vi "DB - [CMS].[Config].[WindowView].vi"(0 "connection reference":T3, 1 "DB Connection":T4={"Open"=TRUE, "Close"=TRUE}, 2 "DB - CMS Config View":T2, 3 "<Values>":string[](array[string])=["Seq 1/2: +150°C/hr to 80°C"], 5 "DB.Schema.Table\nCMS.Config.View":string="CMS.Config.View", 9 "[PlantId],[StationId]":T1, 11 "error in (no error)":errorcluster) -> (4 "connection reference":T3, 6 "data":string[][](array[string]), 15 "SUMMARY":errorcluster)   [LabVIEW 2013]
uses:
  <vilib>/addons/database/Connection.llb/Conn ObjectReference.ctl
  Controls/DB - OpenClose.ctl
  Controls/DB - CMS Config WindowView.ctl
  Controls/Global SRTRS.vi
  Controls/Global CMS.vi
  <vilib>/addons/database/Connection.llb/DB Tools Open Connec (String).vi
  <vilib>/addons/database/Connection.llb/Conn Execute.vi
  <vilib>/addons/database/Recordset.llb/Rec Fetch Recordset Data (R).vi
  <vilib>/addons/database/Recordset.llb/Rec Destroy - Connection.vi
  <vilib>/addons/database/NI_Database_API.lvlib
panel:
  in  "DB.Schema.Table\nCMS.Config.Station":string="CMS.Config.Station"
  out "Close":errorcluster
  out "SQL Statement":string
  in  "DB.Schema.Table \nCMS.Config.WindowView":string="CMS.Config.WindowView"
  out "CMS Connection Information":T5={"Connection "="SQL Server 32bit HPEnvy", "Username"="admin", "Password"="admin123"}
  # "2014-10-21 15:01\n[TabId],                         w.[No],        v.[ToggleTabInterval],w.[ToggleWinInterval], v.[ToggleTab],        v.[DisplayPlant],       w.[Window01],            w.[Window02]"
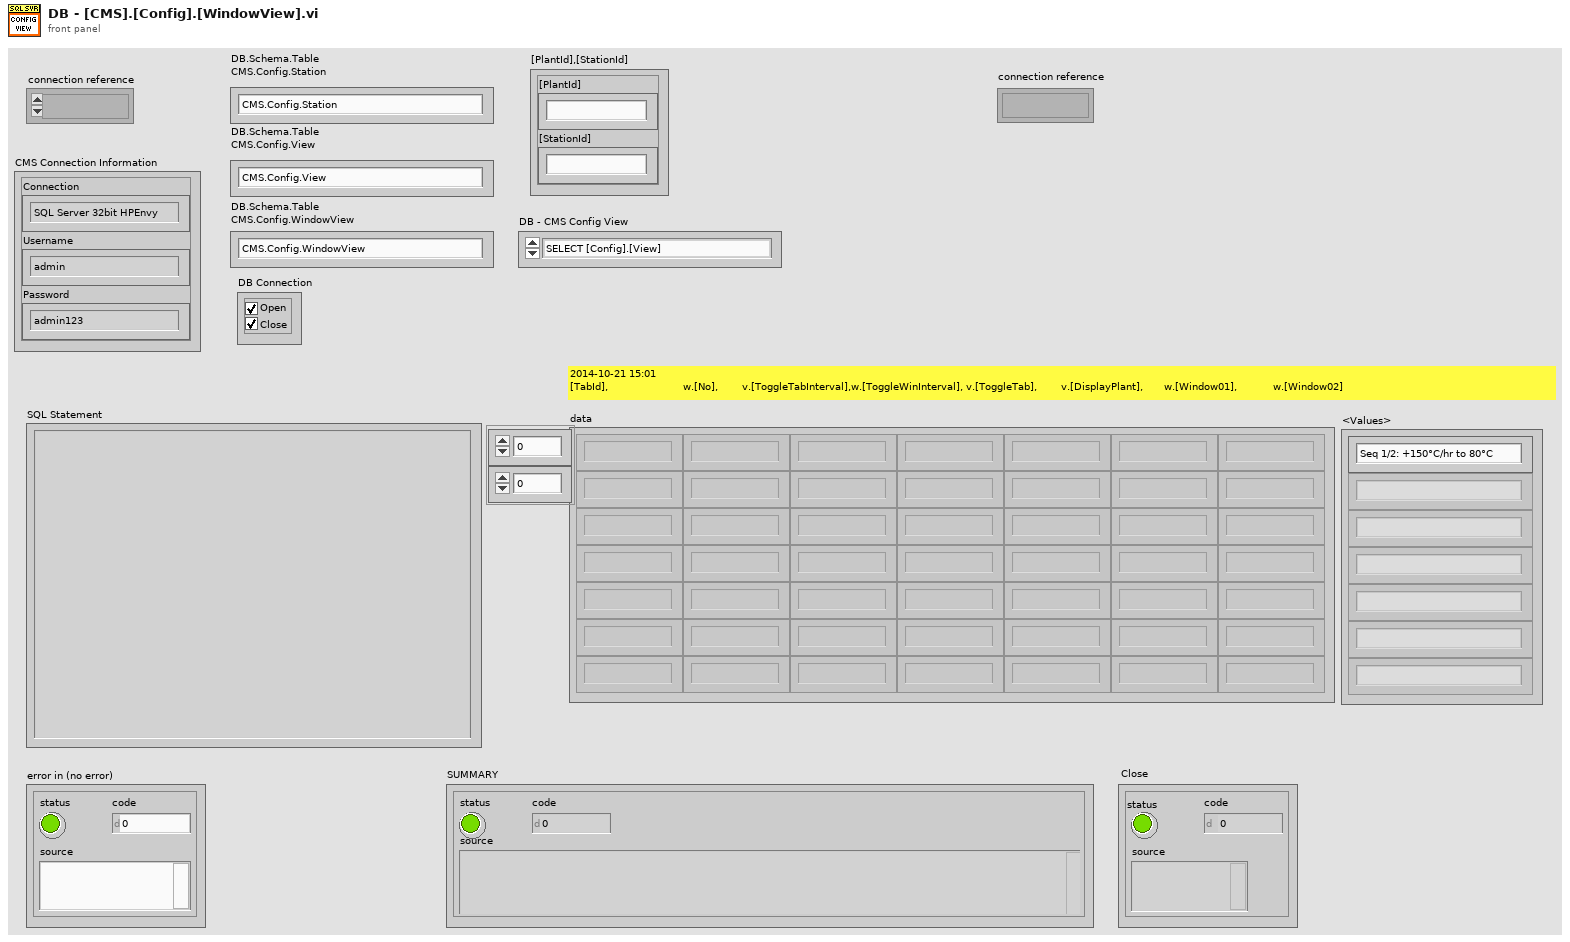
[diagram p1: front panel]
types:
  T1 = cluster{"[PlantId]":string, "[StationId]":string}
  T2 = typedef "DB - CMS Config WindowView.ctl" = enum16{"SELECT [Config].[View]"}
  T3 = typedef "NI_Database_API.lvlib/Conn ObjectReference.ctl" = refnum<k1>
  T4 = typedef "DB - OpenClose.ctl" = cluster{"Open":bool, "Close":bool}
  T5 = cluster{"Connection ":string, "Username":string, "Password":string}
  T6 = typedef "Enum - InteractiveMode-SubVIMode.ctl" = enum16{"Interactive", "subVI Mode"}
  T7 = typedef "DB - DB.Schema.Table.ctl" = cluster{"DB":string, "Schema":string, "Table":string}
  T8 = typedef "Connection Information Cluster.ctl" = cluster{"Connection ":string, "Username":string, "Password":string}
  T9 = typedef "NI_Database_API.lvlib/Rec ObjectReference.ctl" = refnum<k1>
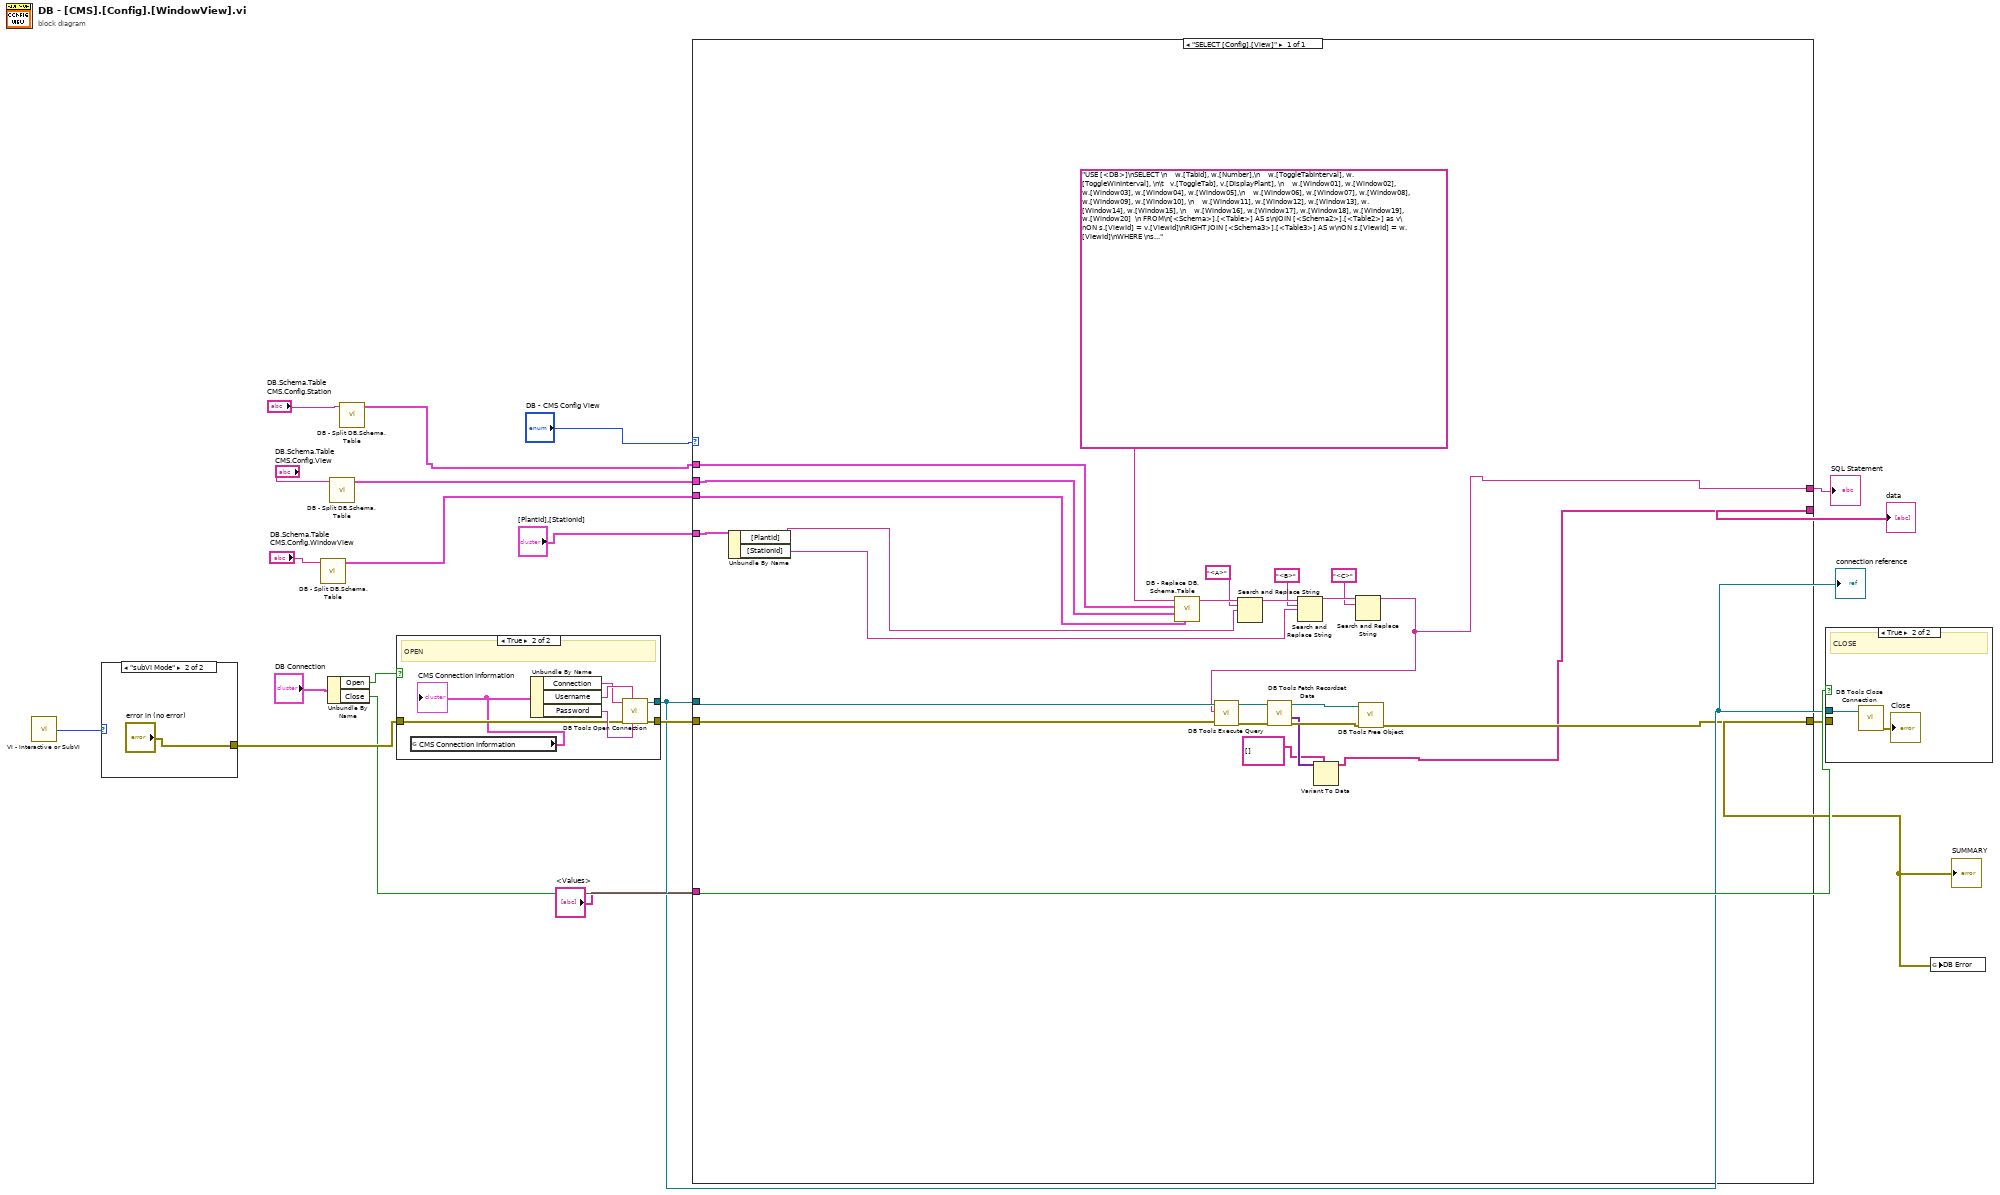
[diagram p0: block diagram]
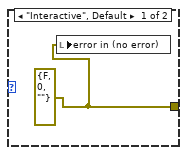
[diagram p3: hidden frame]
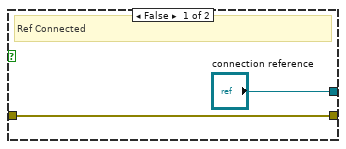
[diagram p4: hidden frame]
diagram:
  n1 = call "VI - Interactive or SubVI.vi"() -> ("Mode"=w17:T6)  [unwired: 5 in]
  n2 = case shown="\"subVI Mode\"" w17 {
    tunnel: [w20 "error in (no error)"] -> w16
    frame "Interactive", Default {
      w20 = errorcluster {"status"=FALSE, "code"=0, "source"=""} ("error in (no error)")
      n3 = local write "error in (no error)"(w20) -> ()
    }
    frame "subVI Mode" {
    }
  }
  n4 = call "DB - Split DB.Schema.Table.vi"("DB.Schema.Table"="DB.Schema.Table \nCMS.Config.WindowView") -> ("DB.Schema.Table"=w3:T7)  [unwired: 10 in]
  n5 = Unbundle By Name("DB Connection") -> ("Open"=w18:bool, "Close"=w14:bool)
  n6 = call "DB - Split DB.Schema.Table.vi"("DB.Schema.Table"="DB.Schema.Table\nCMS.Config.View") -> ("DB.Schema.Table"=w11:T7)  [unwired: 10 in]
  n7 = call "DB - Split DB.Schema.Table.vi"("DB.Schema.Table"="DB.Schema.Table\nCMS.Config.Station") -> ("DB.Schema.Table"=w1:T7)  [unwired: 10 in]
  n8 = case shown="True" w18 {
    tunnel: ["connection reference" w27] -> w7
    tunnel: w16 -> [w22 w26]
    tunnel: [w22 w25] -> w15
    frame False {
      # "Ref Connected"
    }
    frame True {
      # "OPEN"
      n9 = global read "Global CMS.vi" "CMS Connection Information"() -> (w24:T8)
      "CMS Connection Information" <- w24
      n10 = Unbundle By Name(w24) -> ("Connection"=w29:string, "Username"=w30:string, "Password"=w28:string)
      n11 = call-poly <vilib>:"DB Tools Open Connection.vi"("password"=w28, "userID"=w30, "error in (no error)"=w26, "connection information"=w29) -> ("error out"=w25:errorcluster, "connection reference"=w27:T3)  [unwired: 4 in]
    }
  }
  "connection reference" <- w7
  n12 = case shown="\"SELECT [Config].[View]\"" "DB - CMS Config View" {
    tunnel: w7 -> [w41]
    tunnel: w15 -> [w40]
    tunnel: w11 -> [w31]
    tunnel: [w39] -> w10
    tunnel: [w38] -> w9
    tunnel: "<Values>" -> [_]
    tunnel: [w33] -> w5
    tunnel: "[PlantId],[StationId]" -> [w37]
    tunnel: w3 -> [w32]
    tunnel: w1 -> [w36]
    frame "SELECT [Config].[View]" {
      n13 = Unbundle By Name(w37) -> ("[PlantId]"=w35:string, "[StationId]"=w34:string)
      n14 = call "DB - Replace DB.Schema.Table.vi"("DB.Schema.Table 3"=w32, "DB.Schema.Table 2"=w31, "DB.Schema.Table"=w36, "string in"="USE [<DB>]\nSELECT \n    w.[TabId], w.[Number],\n    w.[ToggleTabInterval], w.[ToggleWinInterval], \n\t   v.[ToggleTab], v.[DisplayPlant], \n    w.[Window01], w.[Window02], w.[Window03], w.[Window04], w.[Window05],\n    w.[Window06], w.[Window07], w.[Window08], w.[Window09], w.[Window10], \n    w.[Window11], w.[Window12], w.[Window13], w.[Window14], w.[Window15], \n    w.[Window16], w.[Window17], w.[Window18], w.[Window19], w.[Window20]  \n FROM\n[<Schema>].[<Table>] AS s\nJOIN [<Schema2>].[<Table2>] as v\nON s.[ViewId] = v.[ViewId]\nRIGHT JOIN [<Schema3>].[<Table3>] AS w\nON s.[ViewId] = w.[ViewId]\nWHERE \ns.[PlantId] = '<A>' AND\ns.[StationId] = '<B>' AND\ns.[Inactive] = '0'  AND \nv.[Inactive] = '0'  AND \nw.[Inactive] = '0'\nORDER BY w.[Number] ASC") -> ("string out"=w53:string)  [unwired: 6 in, 1 out]
      n15 = Search and Replace String(input string=w53, search string="<A>", replace string=w35) -> (result string=w51:string)  [unwired: 5 in, 3 out]
      n16 = Search and Replace String(input string=w51, search string="<B>", replace string=w34) -> (result string=w49:string)  [unwired: 5 in, 3 out]
      n17 = Search and Replace String(input string=w49, search string="<C>") -> (result string=w38:string)  [unwired: 6 in, 3 out]
      n18 = call-poly <vilib>:"DB Tools Execute Query.vi"("error in (no error)"=w40, "SQL query"=w38, "connection reference"=w41) -> ("error out"=w45:errorcluster, "recordset reference"=w47:T9)  [unwired: 5 in]
      n19 = call-poly <vilib>:"DB Tools Fetch Recordset Data.vi"("error in (no error)"=w45, "recordset reference"=w47) -> ("error out"=w44:errorcluster, "recordset data"=w43:variant[][], "recordset reference out"=w46:T9)  [unwired: 3 in]
      n20 = Variant To Data(type=string[][] [], Variant=w43) -> (data=w33:string[][])  [unwired: 1 in, 1 out]
      n21 = call-poly <vilib>:"DB Tools Free Object.vi"("error in (no error)"=w44, "recordset reference"=w46) -> ("error out"=w39:errorcluster)  [unwired: 8 in, 1 out]
    }
  }
  "SUMMARY" <- w10
  "SQL Statement" <- w9
  "data" <- w5
  n22 = case shown="True" w14 {
    tunnel: w7 -> [_ w56]
    tunnel: w10 -> [_ _]
    frame False {
      # "Ref Connected"
    }
    frame True {
      # "CLOSE"
      n23 = call <vilib>:"DB Tools Close Connection.vi"("connection reference"=w56) -> ("error out"=→"Close":errorcluster)  [unwired: 6 in]
    }
  }
  n24 = global write "Global SRTRS.vi" "DB Error"(w10) -> ()
